vi "Pick and place sequence.vi"(6 "Component Tray map":T1(array[cluster]), 7 "Assembly Type":string, 8 "error in (no error)":errorcluster, 9 "Assembly Tray map":T1(array[cluster]), 10 "PUT map":T1(array[cluster]), 11 "Assembly Run in":refnum<class "Assembly Run.lvclass">) -> (0 "error out":errorcluster, 3 "Assembly Run out":refnum<class "Assembly Run.lvclass">)   [LabVIEW 2021, in "Assembly Run.lvclass"]
uses:
  Assembly Run.lvclass
  Workspace/Fixture Enum.ctl
  Routine/Routine Enum.ctl
  Workspace/Fixture.lvclass
  Routine/Routine.lvclass
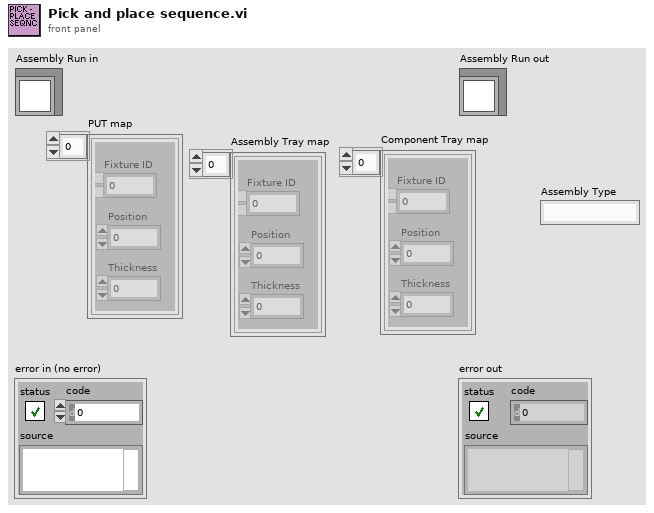
[diagram p1: front panel]
types:
  T1 = cluster{"Fixture ID":dbl, "Position":dbl, "Thickness":dbl}[]
  T2 = typedef "Routine.lvclass/Routine Enum.ctl" = enum16{"Primary Pick Up", "Secondary Pick Up", "Put Down All", "Secure Syringe", "Release Syringe", "Dispense Epoxy", "Pick Up All", "Put Down Secondary", "Full Assembly"}
  T3 = typedef "Fixture.lvclass/Fixture Enum.ctl" = enum16{"Assembly Tray", "Syringe Space", "Component", "Pick Up Tool", "Current Position"}
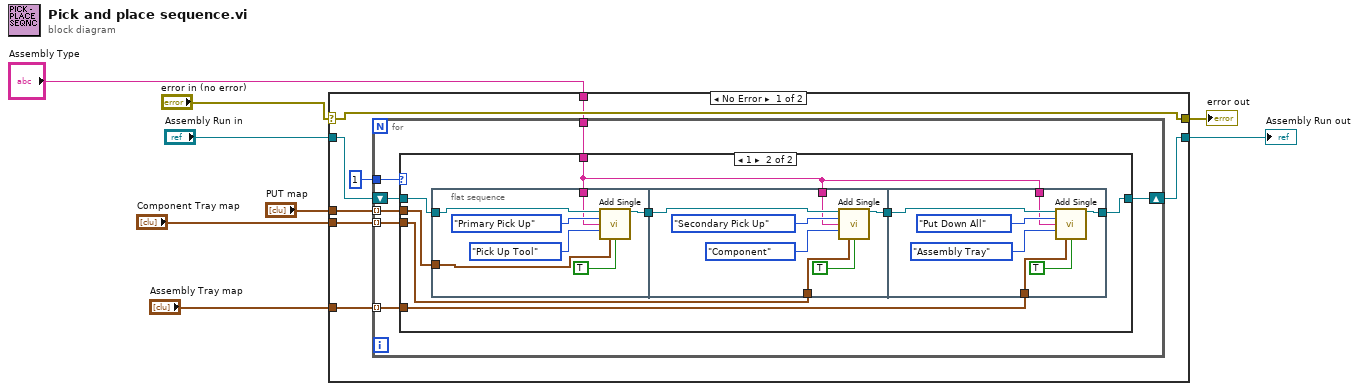
[diagram p0: block diagram]
diagram:
  n1 = case shown="No Error" "error in (no error)" {
    selector: "error in (no error)" -> [w16 w55]
    tunnel: [w16 w55] -> w7
    tunnel: [w13 w54] -> w5
    tunnel: "Assembly Run in" -> [w14 w54]
    tunnel: "PUT map" -> [w12 _]
    tunnel: "Component Tray map" -> [w11 _]
    tunnel: "Assembly Tray map" -> [w10 _]
    tunnel: "Assembly Type" -> [w9 _]
    frame No Error {
      n2 = for {
        tunnel: 1 -> [w21]
        shift-right: [w23] -> w13
        shift-left: w14 -> [w22]
        tunnel: w12 -> [w20] mode=indexing
        tunnel: w11 -> [w19] mode=indexing
        tunnel: w10 -> [w18] mode=indexing
        tunnel: w9 -> [w17]
        n3 = case shown="1" w21 {
          tunnel: [w24 w32] -> w23
          tunnel: w22 -> [w24 w31]
          tunnel: w20 -> [_ w28]
          tunnel: w19 -> [_ w27]
          tunnel: w18 -> [_ w26]
          tunnel: w17 -> [_ w25]
          frame 0, Default {
          }
          frame 1 {
            n4 = flat-sequence {
              tunnel: w31 -> [w38]
              tunnel: [w39] -> w30
              tunnel: w28 -> [w35]
              tunnel: w25 -> [w33]
              tunnel: w30 -> [w46]
              tunnel: [w45] -> w29
              tunnel: w27 -> [w44]
              tunnel: w25 -> [w40]
              tunnel: [w52] -> w32
              tunnel: w29 -> [w53]
              tunnel: w26 -> [w51]
              tunnel: w25 -> [w47]
              frame #0 {
                n5 = call-dynamic "Add Single.vi"("UI in"=w38, "Routine"=Routine_Enum."Primary Pick Up" ("Routine 2"), "Assembly Type"=w33, "Fixture"=Fixture_Enum."Pick Up Tool", "Input Settings"=w35, "Auto"=TRUE) -> ("UI out"=w39:refnum<class "Assembly Run.lvclass">)  [unwired: 8 in, 1 out]
              }
              frame #1 {
                n6 = call-dynamic "Add Single.vi"("UI in"=w46, "Routine"=Routine_Enum."Secondary Pick Up" ("Routine 2"), "Assembly Type"=w40, "Fixture"=Fixture_Enum."Component", "Input Settings"=w44, "Auto"=TRUE) -> ("UI out"=w45:refnum<class "Assembly Run.lvclass">)  [unwired: 8 in, 1 out]
              }
              frame #2 {
                n7 = call-dynamic "Add Single.vi"("UI in"=w53, "Routine"=Routine_Enum."Put Down All" ("Routine 2"), "Assembly Type"=w47, "Fixture"=Fixture_Enum."Assembly Tray", "Input Settings"=w51, "Auto"=TRUE) -> ("UI out"=w52:refnum<class "Assembly Run.lvclass">)  [unwired: 8 in, 1 out]
              }
            }
          }
        }
      }
    }
    frame Error {
    }
  }
  "error out" <- w7
  "Assembly Run out" <- w5
